vi "Read T3110.vi"(8 "error in":errorcluster, 11 "Modbus master in":refnum<class "Modbus Master.lvclass">) -> (0 "error out":errorcluster, 2 "Humidity, %":dbl format="%#_1g", 3 "Temperature, deg C":dbl format="%#_1g")   [LabVIEW 2014, in "T3110 & T2114.lvlib"]
uses:
  T3110 & T2114.lvlib
  <vilib>/NI/Modbus Library/API/Master/Modbus Master.lvclass
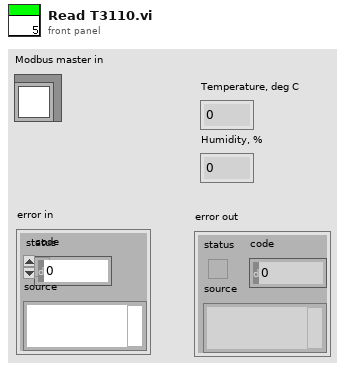
[diagram p1: front panel]
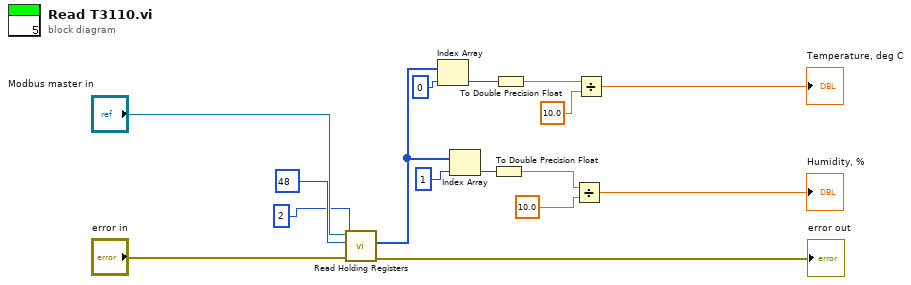
[diagram p0: block diagram]
diagram:
  n1 = call-dynamic "Read Holding Registers.vi"("error in"="error in", "number of inputs"=u16 2, "starting address"=u16 48, "Modbus master in"="Modbus master in") -> ("error out"=→"error out":errorcluster, "register values"=w14:u16[])  [unwired: 5 in, 1 out]
  n2 = Index Array(array=w14, index=0) -> (element=w11:u16)
  n3 = Index Array(array=w14, index=1) -> (element=w10:u16)
  n4 = To Double Precision Float(number=w10) -> (double precision float=w7:dbl)
  n5 = To Double Precision Float(number=w11) -> (double precision float=w9:dbl)
  n6 = Divide(x=w7, y=10.0) -> (x/y=→"Humidity, %":dbl)
  n7 = Divide(x=w9, y=10.0) -> (x/y=→"Temperature, deg C":dbl)
